vi "MuxController.vi"() -> ()   [LabVIEW 2019]
uses:
  <vilib>/rvi/interface/nirviOpenFPGA/nirviOpenFPGA.xnode
  <vilib>/FPGA/interface/niFpgaViExecutionMode.ctl
  <vilib>/rvi/interface/nirviMethod/nirviMethod.xnode
  FPGA Bitfiles/muxcontroller_FPGATarget_DAQmx_WN2VLmabpaE.lvbitx
  DAQmx.vi
  <vilib>/FPGAPlugInAG/PCIe-7842R/niLvFpga_StartFifo_PCIe-7842R.vi
  <vilib>/rvi/errors/niLvFpgaMergeErrorWithErrorCode.vi
  <vilib>/rvi/interface/nirviCloseFPGA/nirviCloseFPGA.xnode
  <vilib>/FPGAPlugInAG/PCIe-7842R/niLvFpga_Close_PCIe-7842R.vi
  <vilib>/rvi/interface/nirviReadWriteControl/nirviReadWriteControl.xnode
  <vilib>/FPGAPlugInAG/PCIe-7842R/niLvFpga_Open_PCIe-7842R.vi
  <vilib>/FPGAPlugInAG/PCIe-7842R/niLvFpga_Reset_PCIe-7842R.vi
  NiFpgaLv.dll
  <vilib>/Utility/error.llb/Error Cluster From Error Code.vi
  <vilib>/rvi/errors/niLvFpgaAdjustHostInterfaceError.vi
  <vilib>/FPGAPlugInAG/PCIe-7842R/niLvFpga_Run_PCIe-7842R.vi
  <vilib>/FPGAPlugInAG/PCIe-7842R/niLvFpga_ReadFifo_PCIe-7842R.vi
  <vilib>/FPGAPlugInAG/PCIe-7842R/niLvFpga_WriteFifo_PCIe-7842R.vi
panel:
  out "Waveform Chart":i16[](graph)
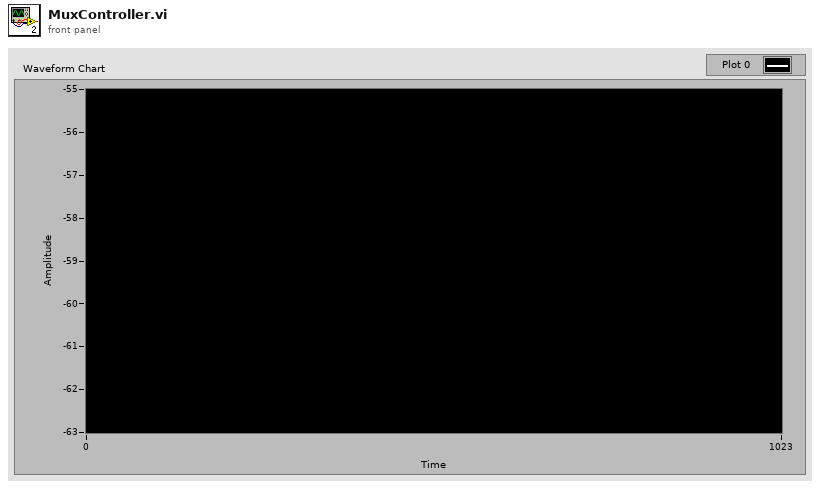
[diagram p1: front panel]
types:
  T1 = typedef "niFpgaViExecutionMode.ctl" = enum16{"FPGA Target", "Simulation (Simulated I/O)", "Simulation (Real I/O)", "Third-Party Simulation"}
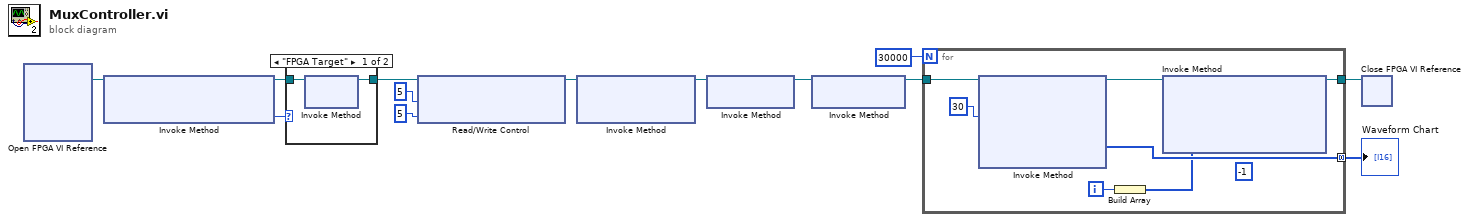
[diagram p0: block diagram]
diagram:
  n1 = xnode "Open FPGA VI Reference"() -> ("FPGA VI Reference Out"=w13:refnum<k20>)  [unwired: 2 in, 1 out]
  n2 = xnode "Invoke Method"("FPGA VI Reference In"=w13) -> ("FPGA VI Reference Out"=w12:refnum<k20>, "FPGA VI Execution Mode"=w11:T1)  [unwired: 1 in, 1 out]
  n3 = case shown="\"FPGA Target\"" w11 {
    tunnel: w12 -> [w15 w16]
    tunnel: [w14 w16] -> w6
    frame "FPGA Target" {
      n4 = xnode "Invoke Method"("FPGA VI Reference In"=w15) -> ("FPGA VI Reference Out"=w14:refnum<k20>)  [unwired: 1 in, 1 out]
    }
    frame "Simulation (Simulated I/O)", Default {
    }
  }
  n5 = xnode "Read/Write Control"("FPGA VI Reference In"=w6, "AI Count(uSec)"=u32 5, "AO Count(uSec)"=u32 5) -> ("FPGA VI Reference Out"=w5:refnum<k20>)  [unwired: 1 in, 1 out]
  n6 = xnode "Invoke Method"("FPGA VI Reference In"=w5) -> ("FPGA VI Reference Out"=w4:refnum<k20>)  [unwired: 2 in, 1 out]
  n7 = xnode "Invoke Method"("FPGA VI Reference In"=w4) -> ("FPGA VI Reference Out"=w8:refnum<k20>)  [unwired: 1 in, 1 out]
  n8 = xnode "Invoke Method"("FPGA VI Reference In"=w8) -> ("FPGA VI Reference Out"=w3:refnum<k20>)  [unwired: 1 in, 1 out]
  n9 = for {
    N: 30000 -> [_]
    tunnel: [w22] -> w9 mode=concatenating
    tunnel: w3 -> [w23]
    tunnel: [w18] -> w7
    i -> [w20]
    (unwired) -1 ("Timeout")
    n10 = xnode "Invoke Method"("FPGA VI Reference In"=w23, "Number of Elements"=u32 30) -> ("FPGA VI Reference Out"=w21:refnum<k20>, "Data"=w22:i16[])  [unwired: 2 in, 2 out]
    n11 = Build Array(w20) -> (w19:i32[])
    n12 = xnode "Invoke Method"("FPGA VI Reference In"=w21, "Data"=w19) -> ("FPGA VI Reference Out"=w18:refnum<k20>)  [unwired: 2 in, 2 out]
  }
  "Waveform Chart" <- w9
  n13 = xnode "Close FPGA VI Reference"("FPGA VI Reference In"=w7) -> ()  [unwired: 1 in, 1 out]
